vi "error_log.vi"(9 "error":errorcluster) -> ()   [LabVIEW 2013]
uses:
  Global.vi
  <vilib>/Utility/file.llb/Write To Spreadsheet File (string).vi
panel:
  out "Output":path[](array[path])
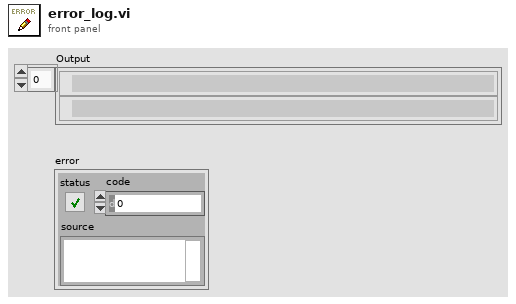
[diagram p1: front panel]
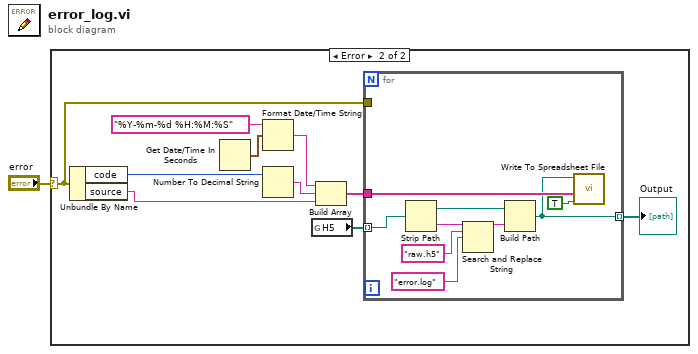
[diagram p0: block diagram]
diagram:
  n1 = case shown="Error" "error" {
    selector: "error" -> [_ w7]
    frame No Error {
    }
    frame Error {
      n2 = Unbundle By Name(w7) -> ("code"=w6:i32, "source"=w3:string)
      n3 = Get Date/Time In Seconds() -> (seconds since 1Jan1904=w8:timestamp)
      n4 = Format Date/Time String(time format string (%c)="%Y-%m-%d %H:%M:%S", seconds (now)=w8) -> (date/time string=w4:string)  [unwired: 1 in]
      n5 = Number To Decimal String(number=w6) -> (decimal integer string=w5:string)  [unwired: 1 in]
      n6 = global read "Global.vi" "H5"() -> (w11:path[])
      n7 = Build Array(w4, w5, w3) -> (w2:string[])
      n8 = for {
        tunnel: w11 -> [w20] mode=indexing
        tunnel: [w12] -> w10 mode=indexing
        tunnel: w7 -> [_]
        tunnel: w2 -> [w13]
        n9 = Strip Path(path=w20) -> (stripped path=w19:path, name=w18:string)
        n10 = Search and Replace String(input string=w18, search string="raw.h5", replace string="error.log" ("replace string (\"\")")) -> (result string=w15:string)  [unwired: 5 in, 3 out]
        n11 = Build Path(base path=w19, name or relative path=w15) -> (appended path=w12:path)
        n12 = call-poly <vilib>:"Write To Spreadsheet File.vi"("append to file? (new file:F)"=TRUE, "1D data"=w13, "file path (dialog if empty)"=w12) -> ()  [unwired: 5 in, 1 out]
      }
      "Output" <- w10
    }
  }
